vi "[Challenge] Condition Based on Measurement Result with Running Total.vi"() -> ()   [LabVIEW 2019]
uses:
  <vilib>/DAQmx/read.llb/DAQmx Read (Analog Wfm 1Chan NSamp).vi
  <vilib>/DAQmx/create/channels.llb/DAQmx Create Channel (AI-Temperature-Thermocouple).vi
  <vilib>/DAQmx/configure/timing.llb/DAQmx Timing (Sample Clock).vi
  <vilib>/DAQmx/miscellaneous.llb/DAQmx Fill In Error Info.vi
  <resource>/objmgr/daqmx.rc
panel:
  in  "Stop":bool
  out "Number of Times Exceeded":i32
  out "Actual Sample Rate (Hz)":dbl
  in  "DAQmx Physical Channel":tag="PCI-6221/ai1"
  out "Last exceeded temperature":waveform(dbl)(graph)={"t0"=timestamp(3640236029.6826963 s since 1904-01-01), "dt"=0.00039059999999999995, "Y"=array[256 elements], "attributes"=variant("NI_ChannelName"=variant(string "PCI-6221/ai0"), "NI_UnitDescription"=variant(string "Deg C"))}
  out "Current temperature":waveform(dbl)(graph)={"t0"=timestamp(3640236029.6826963 s since 1904-01-01), "dt"=0.00039059999999999995, "Y"=array[256 elements], "attributes"=variant("NI_ChannelName"=variant(string "PCI-6221/ai0"), "NI_UnitDescription"=variant(string "Deg C"))}
  in  "Temperature threshold (C)":dbl=50.0
  in  "Number of Samples":i32=256
  in  "Desired Sample Rate (Hz)":dbl=2560.0
  # "Channel Settings"
  # "______________________________________________"
  # "Timing Settings"
  # "______________________________________________"
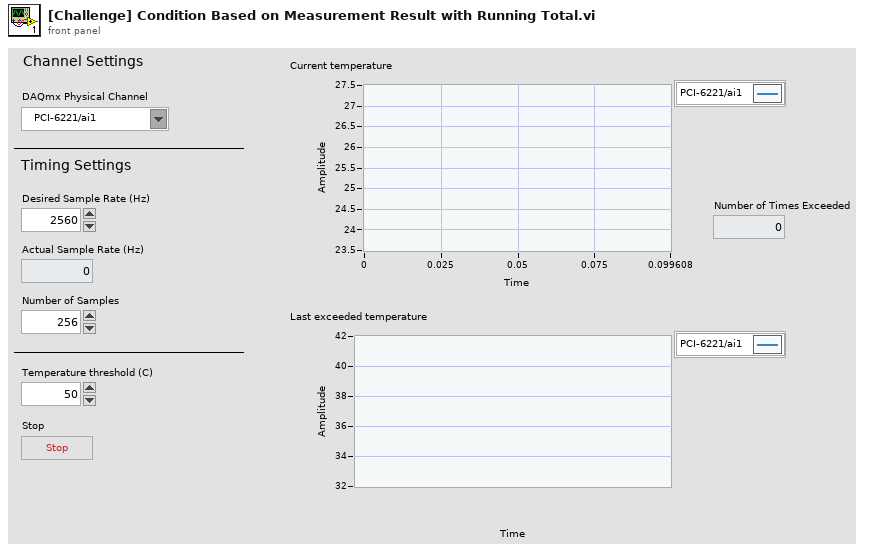
[diagram p1: front panel]
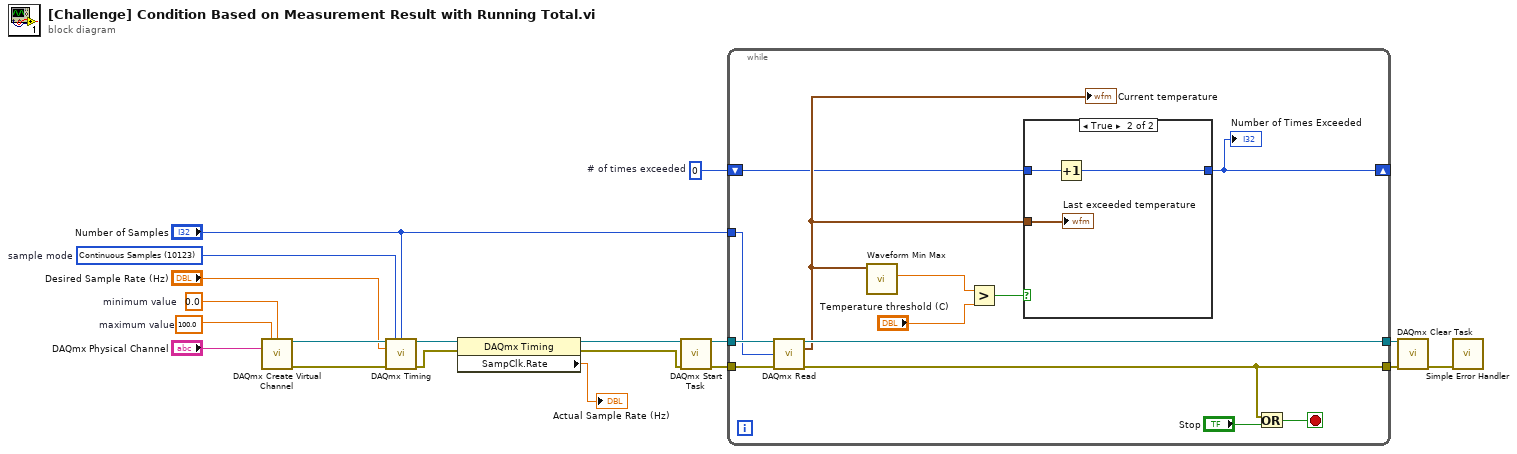
[diagram p0: block diagram]
diagram:
  w1 = 0  # # of times exceeded
  w9 = 100.0  # maximum value
  w10 = 0.0  # minimum value
  w11 = 10123 items=["Finite Samples"=10178, "Continuous Samples"=10123, "Hardware Timed Single Point"=12522]  # sample mode
  n1 = call-poly <vilib>:"DAQmx Create Virtual Channel.vi"("maximum value"=w9, "minimum value"=w10, "physical channels"="DAQmx Physical Channel") -> ("task out"=w19:refnum<k21>, "error out"=w18:errorcluster)  [unwired: 11 in]
  n2 = call-poly <vilib>:"DAQmx Timing.vi"("task/channels in"=w19, "sample mode"=w11, "samples per channel"="Number of Samples", "rate"="Desired Sample Rate (Hz)", "error in"=w18) -> ("task out"=w16:refnum<k21>, "error out"=w17:errorcluster)  [unwired: 9 in]
  n3 = property class="DAQmx Timing"(reference=w16, error in=w17) -> (reference out=w15:refnum<k21>, error out=w14:errorcluster, "SampClk.Rate"=→"Actual Sample Rate (Hz)":dbl)
  n4 = call <vilib>:"DAQmx Start Task.vi"("task/channels in"=w15, "error in"=w14) -> ("task out"=w13:refnum<k21>, "error out"=w12:errorcluster)  [unwired: 12 in]
  n5 = while {
    tunnel: w13 -> [w32]
    tunnel: w12 -> [w31]
    tunnel: "Number of Samples" -> [w23]
    tunnel: [w30] -> w8
    tunnel: [w29] -> w7
    shift-right: [w21] -> _
    shift-left: w1 -> [w22]
    stop <- w28 stop-if-true
    n6 = call-poly <vilib>:"DAQmx Read.vi"("task/channels in"=w32, "number of samples per channel"=w23, "error in"=w31) -> ("task out"=w30:refnum<k21>, "data"=w24:waveform(dbl), "error out"=w29:errorcluster)  [unwired: 10 in]
    "Current temperature" <- w24
    n7 = call <vilib>:"Waveform Min Max.vi"("waveform in"=w24) -> ("Y max"=w27:dbl)  [unwired: 5 in, 5 out]
    n8 = Greater?(x=w27, y="Temperature threshold (C)") -> (0:w26:bool)
    n9 = case shown="True" w26 {
      tunnel: w24 -> [_ w36]
      tunnel: w22 -> [w33 w35]
      tunnel: [w33 w34] -> w21
      frame False {
      }
      frame True {
        n10 = Increment(x=w35) -> (x+1=w34:i32)
        "Last exceeded temperature" <- w36
      }
    }
    "Number of Times Exceeded" <- w21
    n11 = Or(x=w29, y="Stop") -> (x .or. y?=w28:bool)
  }
  n12 = call <vilib>:"DAQmx Clear Task.vi"("task in"=w8, "error in"=w7) -> ("error out"=w6:errorcluster)  [unwired: 13 in]
  n13 = call <vilib>:"Simple Error Handler.vi"("error in (no error)"=w6) -> ()  [unwired: 4 in, 5 out]
